vi "Signal Parameters FG.vi"(7 "Action":T1, 8 "error in (no error)":errorcluster, 10 "Signal Parameters":T2 {"Byte Order" items=["Little Endian", "Big Endian"]; "Data Type" items=["Signed", "Unsigned", "IEEE Float"]}, 11 "Device Item Ref in":T3 format="%.0x") -> (0 "error out":errorcluster, 2 "Signal Parameters":T2 {"Byte Order" items=["Little Endian", "Big Endian"]; "Data Type" items=["Signed", "Unsigned", "IEEE Float"]}, 3 "Device Item Ref out":T3=18446744073709551615 format="%.0x")   [LabVIEW 2015, in "Diagnostics Addon System Explorer.lvlib"]
uses:
  Diagnostics Addon System Explorer.lvlib
  <vilib>/NI Veristand/Custom Device API/Custom Device Item Ref.ctl
  Shared/Types/Signal Parameters.ctl
  Types/FG Action.ctl
  <vilib>/NI Veristand/Custom Device API/Get Item Property (String).vi
  <vilib>/NI Veristand/Custom Device API/Get Item Property (Double).vi
  <vilib>/NI Veristand/Custom Device API/Get Item Property (U32).vi
  <vilib>/NI Veristand/Custom Device API/Set Item Property (String).vi
  <vilib>/NI Veristand/Custom Device API/Set Item Property (Double).vi
  <vilib>/NI Veristand/Custom Device API/Set Item Property (U32).vi
  Shared/SubVIs/GUID Lookup.vi
  Shared/Diagnostics Addon Shared.lvlib
  <vilib>/NI Veristand/Custom Device API/Custom Device API.lvlib
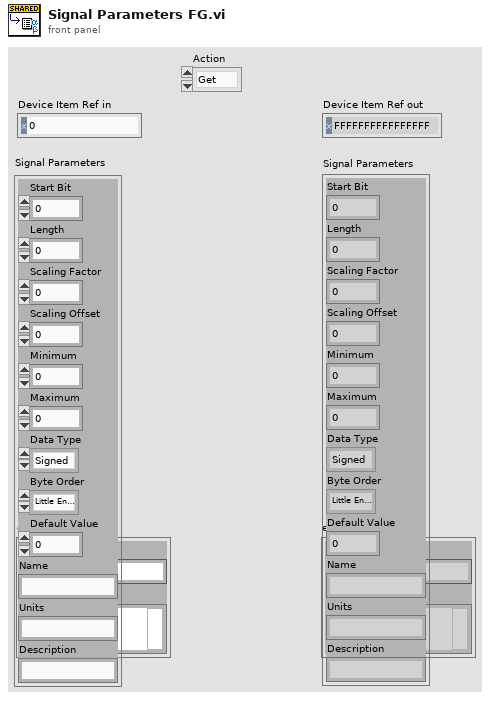
[diagram p1: front panel]
types:
  T1 = typedef "Diagnostics Addon System Explorer.lvlib/FG Action.ctl" = enum16{"Get", "Set"}
  T2 = typedef "Diagnostics Addon Shared.lvlib/Signal Parameters.ctl" = cluster{"Start Bit":u8, "Length":u8, "Scaling Factor":dbl, "Scaling Offset":dbl, "Minimum":dbl, "Maximum":dbl, "Data Type":u32, "Byte Order":u32, "Default Value":dbl, "Name":string, "Units":string, "Description":string}
  T3 = typedef "Custom Device API.lvlib/Custom Device Item Ref.ctl" = u64
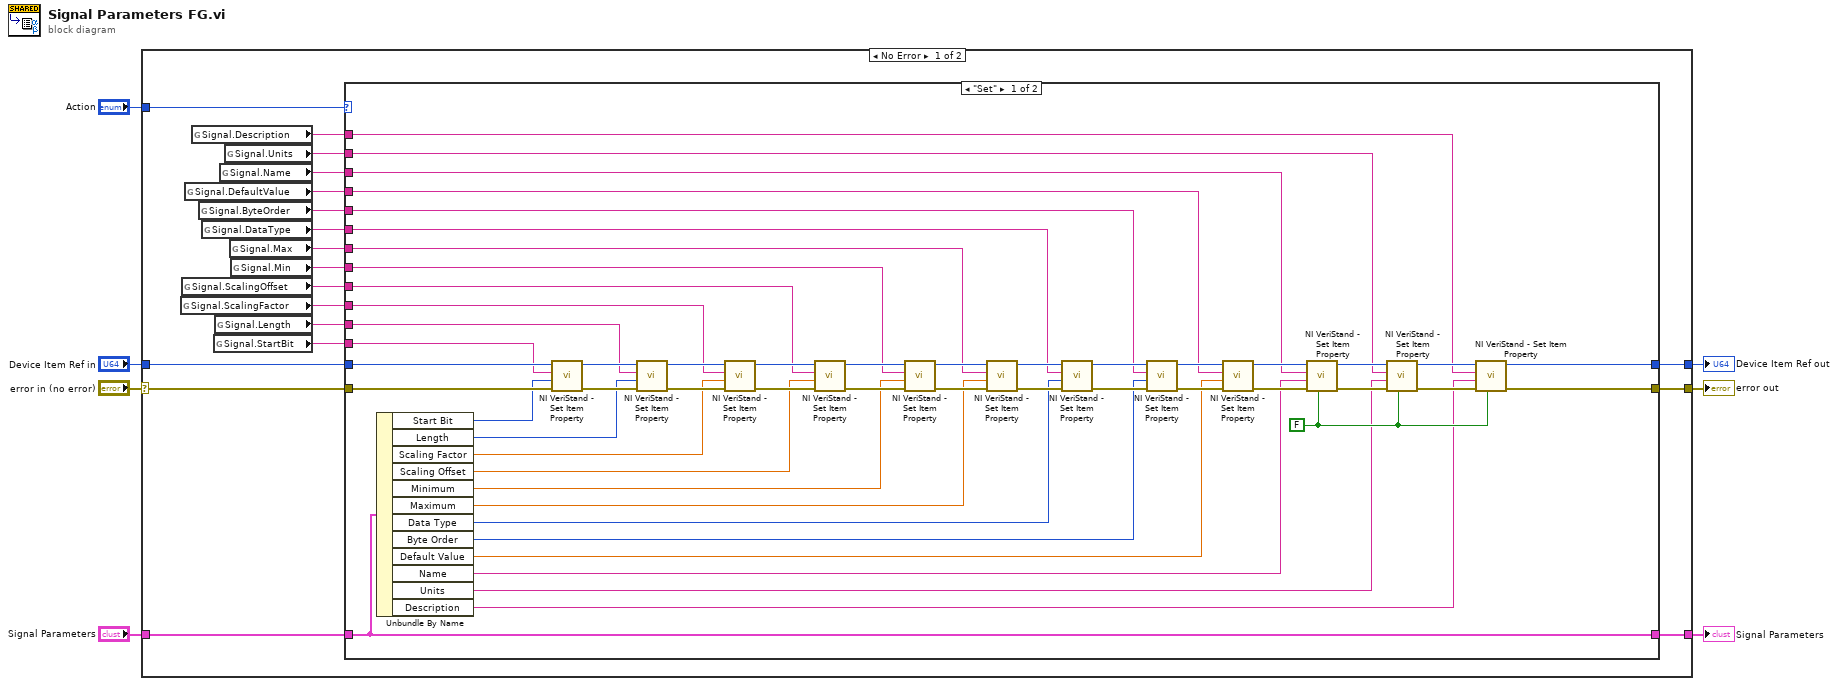
[diagram p0: block diagram]
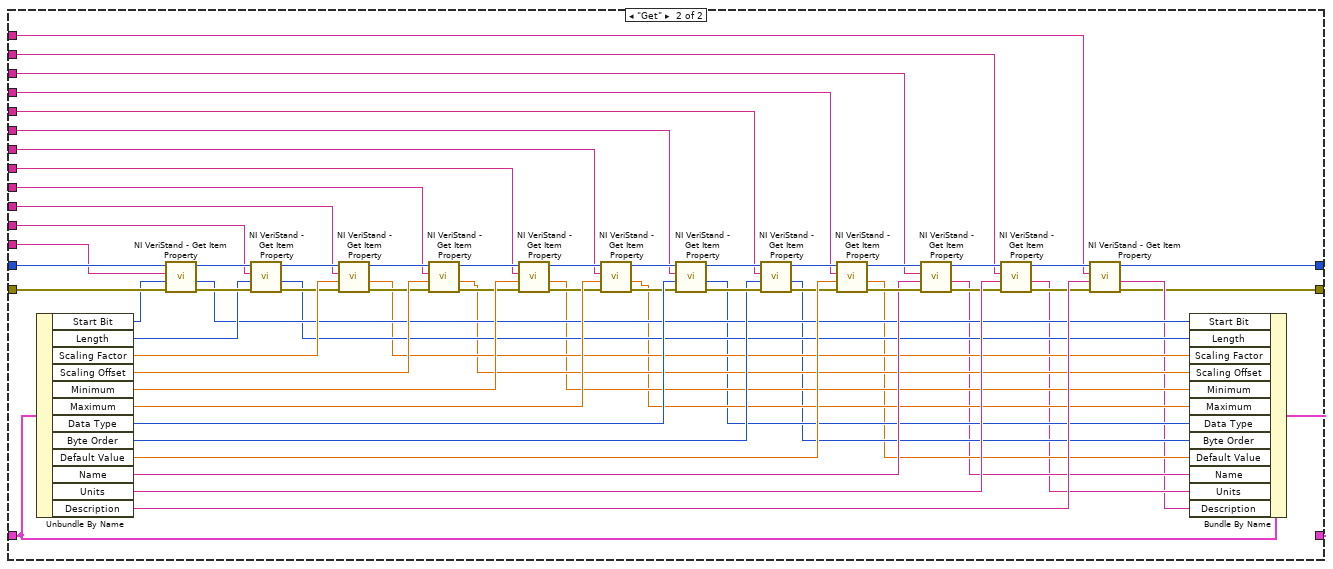
[diagram p2: hidden frame]
diagram:
  n1 = case shown="No Error" "error in (no error)" {
    selector: "error in (no error)" -> [w26 w143]
    tunnel: "Device Item Ref in" -> [w25 w144]
    tunnel: [w24 w144] -> w4
    tunnel: [w23 w143] -> w5
    tunnel: [w22 _] -> w3
    tunnel: "Signal Parameters" -> [w21 _]
    tunnel: "Action" -> [w20 _]
    frame No Error {
      n2 = global read "GUID Lookup.vi" "Signal.ScalingFactor"() -> (w17:string)
      n3 = global read "GUID Lookup.vi" "Signal.ScalingOffset"() -> (w16:string)
      n4 = global read "GUID Lookup.vi" "Signal.DefaultValue"() -> (w11:string)
      n5 = global read "GUID Lookup.vi" "Signal.Description"() -> (w8:string)
      n6 = global read "GUID Lookup.vi" "Signal.ByteOrder"() -> (w12:string)
      n7 = global read "GUID Lookup.vi" "Signal.DataType"() -> (w13:string)
      n8 = global read "GUID Lookup.vi" "Signal.StartBit"() -> (w19:string)
      n9 = global read "GUID Lookup.vi" "Signal.Length"() -> (w18:string)
      n10 = global read "GUID Lookup.vi" "Signal.Name"() -> (w10:string)
      n11 = global read "GUID Lookup.vi" "Signal.Units"() -> (w9:string)
      n12 = global read "GUID Lookup.vi" "Signal.Max"() -> (w14:string)
      n13 = global read "GUID Lookup.vi" "Signal.Min"() -> (w15:string)
      n14 = case shown="\"Set\"" w20 {
        tunnel: w26 -> [w66 w142]
        tunnel: w25 -> [w63 w141]
        tunnel: [w51 w79] -> w24
        tunnel: [w65 w81] -> w23
        tunnel: [w67 w80] -> w22
        tunnel: w21 -> [w67 w94]
        tunnel: w19 -> [w27 w107]
        tunnel: w18 -> [w28 w106]
        tunnel: w17 -> [w29 w105]
        tunnel: w16 -> [w30 w104]
        tunnel: w15 -> [w31 w103]
        tunnel: w14 -> [w32 w102]
        tunnel: w13 -> [w33 w101]
        tunnel: w12 -> [w34 w100]
        tunnel: w11 -> [w35 w99]
        tunnel: w10 -> [w36 w97]
        tunnel: w9 -> [w37 w96]
        tunnel: w8 -> [w38 w95]
        frame "Set" {
          w64 = FALSE ("Binary String (T)")
          n15 = Unbundle By Name(w67) -> ("Start Bit"=w50:u8, "Length"=w49:u8, "Scaling Factor"=w48:dbl, "Scaling Offset"=w47:dbl, "Minimum"=w46:dbl, "Maximum"=w45:dbl, "Data Type"=w44:u32, "Byte Order"=w43:u32, "Default Value"=w42:dbl, "Name"=w41:string, "Units"=w40:string, "Description"=w39:string)
          n16 = call-poly <vilib>:"NI VeriStand - Set Item Property.vi"("error in (no error)"=w66, "Value"=w50, "Property Name"=w27, "Item Ref in"=w63) -> ("error out"=w78:errorcluster, "Item Ref out"=w62:T3)  [unwired: 5 in, 1 out]
          n17 = call-poly <vilib>:"NI VeriStand - Set Item Property.vi"("error in (no error)"=w78, "Value"=w49, "Property Name"=w28, "Item Ref in"=w62) -> ("error out"=w76:errorcluster, "Item Ref out"=w61:T3)  [unwired: 5 in, 1 out]
          n18 = call-poly <vilib>:"NI VeriStand - Set Item Property.vi"("error in (no error)"=w76, "Value"=w48, "Property Name"=w29, "Item Ref in"=w61) -> ("error out"=w75:errorcluster, "Item Ref out"=w60:T3)  [unwired: 5 in, 1 out]
          n19 = call-poly <vilib>:"NI VeriStand - Set Item Property.vi"("error in (no error)"=w75, "Value"=w47, "Property Name"=w30, "Item Ref in"=w60) -> ("error out"=w74:errorcluster, "Item Ref out"=w59:T3)  [unwired: 5 in, 1 out]
          n20 = call-poly <vilib>:"NI VeriStand - Set Item Property.vi"("error in (no error)"=w74, "Value"=w46, "Property Name"=w31, "Item Ref in"=w59) -> ("error out"=w73:errorcluster, "Item Ref out"=w58:T3)  [unwired: 5 in, 1 out]
          n21 = call-poly <vilib>:"NI VeriStand - Set Item Property.vi"("error in (no error)"=w73, "Value"=w45, "Property Name"=w32, "Item Ref in"=w58) -> ("error out"=w72:errorcluster, "Item Ref out"=w57:T3)  [unwired: 5 in, 1 out]
          n22 = call-poly <vilib>:"NI VeriStand - Set Item Property.vi"("error in (no error)"=w72, "Value"=w44, "Property Name"=w33, "Item Ref in"=w57) -> ("error out"=w77:errorcluster, "Item Ref out"=w56:T3)  [unwired: 5 in, 1 out]
          n23 = call-poly <vilib>:"NI VeriStand - Set Item Property.vi"("error in (no error)"=w77, "Value"=w43, "Property Name"=w34, "Item Ref in"=w56) -> ("error out"=w71:errorcluster, "Item Ref out"=w55:T3)  [unwired: 5 in, 1 out]
          n24 = call-poly <vilib>:"NI VeriStand - Set Item Property.vi"("error in (no error)"=w71, "Value"=w42, "Property Name"=w35, "Item Ref in"=w55) -> ("error out"=w70:errorcluster, "Item Ref out"=w54:T3)  [unwired: 5 in, 1 out]
          n25 = call-poly <vilib>:"NI VeriStand - Set Item Property.vi"("Binary String (T)"=w64, "error in (no error)"=w70, "Value"=w41, "Property Name"=w36, "Item Ref in"=w54) -> ("error out"=w69:errorcluster, "Item Ref out"=w53:T3)  [unwired: 4 in, 1 out]
          n26 = call-poly <vilib>:"NI VeriStand - Set Item Property.vi"("Binary String (T)"=w64, "error in (no error)"=w69, "Value"=w40, "Property Name"=w37, "Item Ref in"=w53) -> ("error out"=w68:errorcluster, "Item Ref out"=w52:T3)  [unwired: 4 in, 1 out]
          n27 = call-poly <vilib>:"NI VeriStand - Set Item Property.vi"("Binary String (T)"=w64, "error in (no error)"=w68, "Value"=w39, "Property Name"=w38, "Item Ref in"=w52) -> ("error out"=w65:errorcluster, "Item Ref out"=w51:T3)  [unwired: 4 in, 1 out]
        }
        frame "Get" {
          n28 = Unbundle By Name(w94) -> ("Start Bit"=w140:u8, "Length"=w126:u8, "Scaling Factor"=w125:dbl, "Scaling Offset"=w124:dbl, "Minimum"=w123:dbl, "Maximum"=w122:dbl, "Data Type"=w121:u32, "Byte Order"=w120:u32, "Default Value"=w119:dbl, "Name"=w98:string, "Units"=w118:string, "Description"=w117:string)
          n29 = call-poly <vilib>:"NI VeriStand - Get Item Property.vi"("error in (no error)"=w142, "Default Value"=w140, "Property Name"=w107, "Item Ref in"=w141) -> ("error out"=w138:errorcluster, "Value"=w93:u32, "Item Ref out"=w139:T3)  [unwired: 4 in, 1 out]
          n30 = call-poly <vilib>:"NI VeriStand - Get Item Property.vi"("error in (no error)"=w138, "Default Value"=w126, "Property Name"=w106, "Item Ref in"=w139) -> ("error out"=w116:errorcluster, "Value"=w92:u32, "Item Ref out"=w137:T3)  [unwired: 4 in, 1 out]
          n31 = call-poly <vilib>:"NI VeriStand - Get Item Property.vi"("error in (no error)"=w116, "Default Value"=w125, "Property Name"=w105, "Item Ref in"=w137) -> ("error out"=w115:errorcluster, "Value"=w91:dbl, "Item Ref out"=w136:T3)  [unwired: 4 in, 1 out]
          n32 = call-poly <vilib>:"NI VeriStand - Get Item Property.vi"("error in (no error)"=w115, "Default Value"=w124, "Property Name"=w104, "Item Ref in"=w136) -> ("error out"=w114:errorcluster, "Value"=w90:dbl, "Item Ref out"=w135:T3)  [unwired: 4 in, 1 out]
          n33 = call-poly <vilib>:"NI VeriStand - Get Item Property.vi"("error in (no error)"=w114, "Default Value"=w123, "Property Name"=w103, "Item Ref in"=w135) -> ("error out"=w113:errorcluster, "Value"=w89:dbl, "Item Ref out"=w134:T3)  [unwired: 4 in, 1 out]
          n34 = call-poly <vilib>:"NI VeriStand - Get Item Property.vi"("error in (no error)"=w113, "Default Value"=w122, "Property Name"=w102, "Item Ref in"=w134) -> ("error out"=w112:errorcluster, "Value"=w88:dbl, "Item Ref out"=w132:T3)  [unwired: 4 in, 1 out]
          n35 = call-poly <vilib>:"NI VeriStand - Get Item Property.vi"("error in (no error)"=w112, "Default Value"=w121, "Property Name"=w101, "Item Ref in"=w132) -> ("error out"=w133:errorcluster, "Value"=w87:u32, "Item Ref out"=w131:T3)  [unwired: 4 in, 1 out]
          n36 = call-poly <vilib>:"NI VeriStand - Get Item Property.vi"("error in (no error)"=w133, "Default Value"=w120, "Property Name"=w100, "Item Ref in"=w131) -> ("error out"=w111:errorcluster, "Value"=w86:u32, "Item Ref out"=w130:T3)  [unwired: 4 in, 1 out]
          n37 = call-poly <vilib>:"NI VeriStand - Get Item Property.vi"("error in (no error)"=w111, "Default Value"=w119, "Property Name"=w99, "Item Ref in"=w130) -> ("error out"=w110:errorcluster, "Value"=w85:dbl, "Item Ref out"=w129:T3)  [unwired: 4 in, 1 out]
          n38 = call-poly <vilib>:"NI VeriStand - Get Item Property.vi"("error in (no error)"=w110, "Default Value"=w98, "Property Name"=w97, "Item Ref in"=w129) -> ("error out"=w109:errorcluster, "Value"=w84:string, "Item Ref out"=w128:T3)  [unwired: 4 in, 1 out]
          n39 = call-poly <vilib>:"NI VeriStand - Get Item Property.vi"("error in (no error)"=w109, "Default Value"=w118, "Property Name"=w96, "Item Ref in"=w128) -> ("error out"=w108:errorcluster, "Value"=w83:string, "Item Ref out"=w127:T3)  [unwired: 4 in, 1 out]
          n40 = call-poly <vilib>:"NI VeriStand - Get Item Property.vi"("error in (no error)"=w108, "Default Value"=w117, "Property Name"=w95, "Item Ref in"=w127) -> ("error out"=w81:errorcluster, "Value"=w82:string, "Item Ref out"=w79:T3)  [unwired: 4 in, 1 out]
          n41 = Bundle By Name(cluster=w94, "Start Bit"=w93, "Length"=w92, "Scaling Factor"=w91, "Scaling Offset"=w90, "Minimum"=w89, "Maximum"=w88, "Data Type"=w87, "Byte Order"=w86, "Default Value"=w85, "Name"=w84, "Units"=w83, "Description"=w82) -> (w80:T2)
        }
      }
    }
    frame Error {
    }
  }
  "error out" <- w5
  "Device Item Ref out" <- w4
  "Signal Parameters" <- w3
